vi "MainDequeue.vi"(8 "エラー入力（エラーなし）":errorcluster, 11 "キュー入力":refnum<queue>) -> (0 "エラー出力":errorcluster, 1 "Data":variant, 2 "StepName":T1, 3 "キュー出力":refnum<queue>)   [LabVIEW 2021]
doc: "SP1TaskLoop および、SP2TaskLoop へのコマンド用キューを受信します。\nキューに入れるデータは、コマンド（StepName）とデータ（Data）の入ったクラスタです。\n列挙隊のコマンド（StepName）とバリアントのデータ（Data）を出力します。"
uses:
  MainStatus.ctl
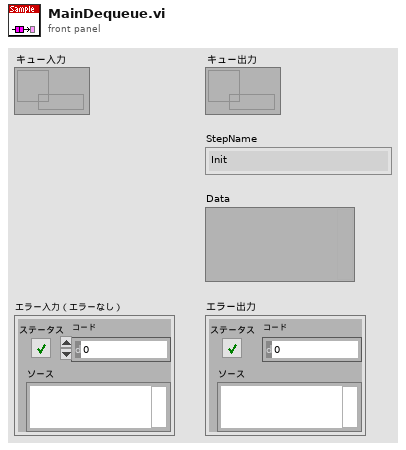
[diagram p1: front panel]
types:
  T1 = typedef "MainStatus.ctl" = enum16{"Init", "Status", "Placed", "Setting", "Start", "Data", "Collected", "Quit"}
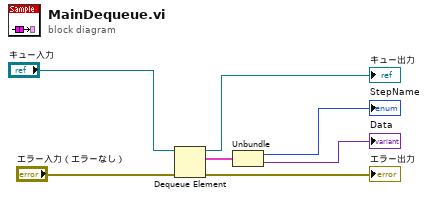
[diagram p0: block diagram]
diagram:
  n1 = Dequeue Element(queue="キュー入力", error in (no error)="エラー入力（エラーなし）") -> (queue out=→"キュー出力":refnum<queue>, element=w3:cluster{"StepName":T1, "Data":variant}, error out=→"エラー出力":errorcluster)  [unwired: 1 in, 1 out]
  n2 = Unbundle(w3) -> ("StepName"=→"StepName":T1, "Data"=→"Data":variant)
